vi "PathPlanner_PointTowardsZone_Flip.vi"(11 "PointTowardsZone":T1={"RotationOffset"={"VALUE"=0.0, "COS"=1.0, "SIN"=0.0}, "Name"="", "TargetPosition"={"X"=0.0, "Y"=0.0}, "MinPosition"=0.0, "MaxPosition"=0.0} {"TargetPosition"."Y" format="%14.3f"; "TargetPosition"."X" format="%14.3f"; "RotationOffset"."SIN" format="%13.4f"; "RotationOffset"."COS" format="%13.4f"; "RotationOffset"."VALUE" format="%13.4f"}) -> (3 "FlippedPointTowardsZone":T1={"RotationOffset"={"VALUE"=0.0, "COS"=1.0, "SIN"=0.0}, "Name"="", "TargetPosition"={"X"=0.0, "Y"=0.0}, "MinPosition"=0.0, "MaxPosition"=0.0} {"TargetPosition"."Y" format="%14.3f"; "TargetPosition"."X" format="%14.3f"; "RotationOffset"."SIN" format="%13.4f"; "RotationOffset"."COS" format="%13.4f"; "RotationOffset"."VALUE" format="%13.4f"})   [LabVIEW 2019, in "PathPlanner24.lvlib"]
doc: "Flip this point towards zone to the other side of the field, maintaining a blue alliance origin\n\nInputs: \n - PointTowardsZone - cluster -- The cluster to flip.\n\nOutputs:\n - FlippedPointTowardsZone - cluster -- The flipped cluster."
uses:
  PathPlanner24.lvlib
  TypeDef/PathPlannerPointTowardsZone.ctl
  <vilib>/Rock Robotics/WPI/ThirdParty/JAS_Junk/TrajLib/TypeDef/ROTATION2D.ctl
  <vilib>/Rock Robotics/WPI/ThirdParty/JAS_Junk/TrajLib/TypeDef/TRANSLATION2D.ctl
  PathPlanner_FieldUtil_SymmetryType.vi
  PathPlanner_FieldUtil_FieldSizeY.vi
  <vilib>/Rock Robotics/WPI/ThirdParty/JAS_Junk/TrajLib/Translation2d_GetXY.vi
  <vilib>/Rock Robotics/WPI/ThirdParty/JAS_Junk/TrajLib/Translation2d_Create.vi
  PathPlanner_FieldUtil_FieldSizeX.vi
  <vilib>/Rock Robotics/WPI/ThirdParty/JAS_Junk/TrajLib/Conv_Feet_Meters.vi
  <vilib>/Rock Robotics/WPI/ThirdParty/JAS_Junk/TrajLib/Trajectory_Library.lvlib
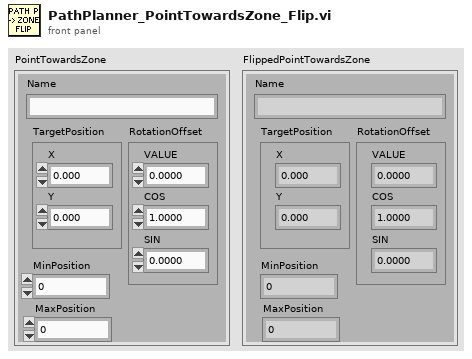
[diagram p1: front panel]
types:
  T1 = typedef "PathPlanner24.lvlib/PathPlannerPointTowardsZone.ctl" = cluster{"RotationOffset":T2, "Name":string, "TargetPosition":T3, "MinPosition":dbl, "MaxPosition":dbl}
  T2 = typedef "Trajectory_Library.lvlib/ROTATION2D.ctl" = cluster{"VALUE":dbl, "COS":dbl, "SIN":dbl}
  T3 = typedef "Trajectory_Library.lvlib/TRANSLATION2D.ctl" = cluster{"X":dbl, "Y":dbl}
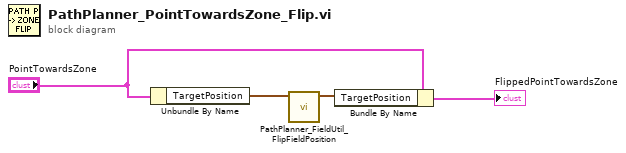
[diagram p0: block diagram]
diagram:
  n1 = Unbundle By Name("PointTowardsZone") -> ("TargetPosition"=w1:T3)
  n2 = call "PathPlanner_FieldUtil_FlipFieldPosition.vi"("FieldPosition"=w1) -> ("FlippedFieldPosition"=w2:T3)  [unwired: 10 in]
  n3 = Bundle By Name(cluster="PointTowardsZone", "TargetPosition"=w2) -> (→"FlippedPointTowardsZone":T1)
